vi "Create Chained Command.vi"(9 "Imported Commands":string[][](array[string]), 10 "String":string) -> (2 "output cluster":T1)   [LabVIEW 2020]
uses:
  Data Cluster.ctl
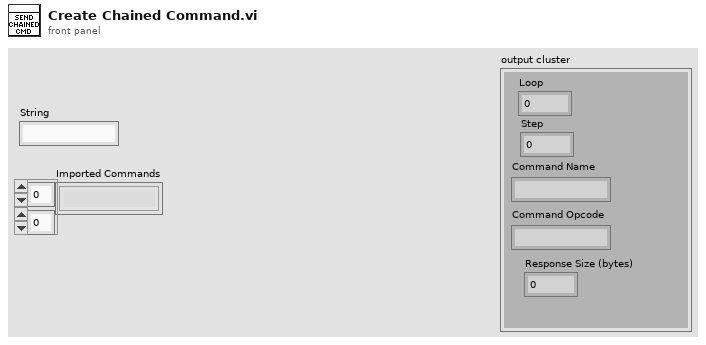
[diagram p1: front panel]
types:
  T1 = typedef "Data Cluster.ctl" = cluster{"Command Name":string, "Command Opcode ":string, "Step":dbl, "Loop":dbl, "Response Size (bytes)":u16}
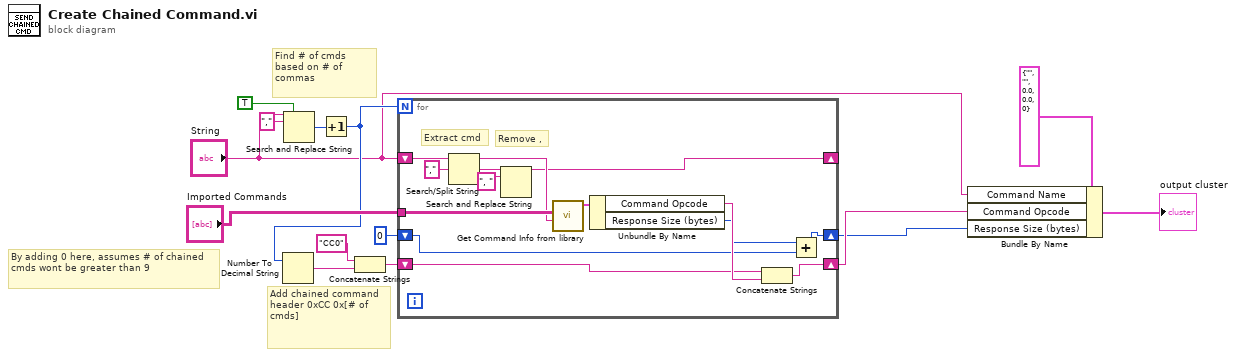
[diagram p0: block diagram]
diagram:
  # "By adding 0 here, assumes # of chained cmds wont be greater than 9"
  # "Add chained command header 0xCC 0x[# of cmds]"
  # "Find # of cmds based on # of commas"
  n1 = Search and Replace String(replace all?=TRUE ("replace all? (F)"), input string="String", search string=",") -> (number of replacements=w8:i32)  [unwired: 5 in, 3 out]
  n2 = Increment(x=w8) -> (x+1=w7:i32)
  n3 = Number To Decimal String(number=w7) -> (decimal integer string=w12:string)  [unwired: 1 in]
  n4 = Concatenate Strings("CC0", w12) -> (w10:string)
  n5 = for {
    N: w7 -> [_]
    tunnel: "Imported Commands" -> [w24]
    shift-right: [w19] -> w5
    shift-left: w10 -> [w20]
    shift-right: [w18] -> _
    shift-left: "String" -> [w25]
    shift-right: [w16] -> w2
    shift-left: 0 -> [w17]
    # "Remove ,"
    # "Extract cmd"
    n6 = Search/Split String(string=w25, search string/char (-)=",") -> (substring before match=w23:string, match + rest of string=w28:string)  [unwired: 1 in, 1 out]
    n7 = Search and Replace String(input string=w28, search string=", ") -> (result string=w18:string)  [unwired: 6 in, 3 out]
    n8 = call "Get Command Info from library.vi"("Step"=w23, "Imported Commands"=w24) -> ("Data cluster"=w22:T1)  [unwired: 9 in]
    n9 = Unbundle By Name(w22) -> ("Command Opcode"=w21:string, "Response Size (bytes)"=w15:u16)
    n10 = Concatenate Strings(w20, w21) -> (w19:string)
    n11 = Add(x=w15, y=w17) -> (x+y=w16:i32)
  }
  n12 = Bundle By Name(cluster=T1 {"Command Name"="", "Command Opcode "="", "Step"=0.0, "Loop"=0.0, "Response Size (bytes)"=0} ("Data Cluster"), "Command Name"="String", "Command Opcode"=w5, "Response Size (bytes)"=w2) -> (→"output cluster":T1)
